vi "Send Control Drag Starting.vi"(0 "Message Enqueuer in":refnum<class "Message Enqueuer.lvclass">, 1 "Drag Mode":enum32{"copy or move", "copy only", "move only"}(ring), 3 "EventFilter Reference":T3, 5 "CtlRef":refnum<vi>, 7 "Time":u32, 9 "Coords":T2, 11 "Button":u16, 12 "Mods":cluster{"Double Click":bool, "Menu Key":bool}, 13 "PlatMods":T4, 14 "Data":T1(array[cluster])) -> (4 "Filtered EventDataMessage":refnum<class "ControlDragStartingMsg.lvclass">, 15 "error out":errorcluster)   [LabVIEW 2020, in "MVA Framework.lvlib" / "ActorEvents.lvlib" / "ControlDragStartingMsg.lvclass"]
doc: "<License>\nCopyright © 2017 Composed Systems, LLC | All rights reserved\nwww.composed.io\n\nAuthor: Ethan Stern <ethan.stern@composed.io>\n\nThis software is provided \"AS IS\" WITHOUT WARRANTIES, either express or implied, AND IS FOR EDUCATIONAL PURPOSES ONLY.\n</License>"
uses:
  ControlDragStartingMsg.lvclass
  <vilib>/ActorFramework/Message Enqueuer/Message Enqueuer.lvclass
  IEventFilter/EventFilter Reference.ctl
  IEventFilter/IEventFilter.lvclass
  <vilib>/Utility/miscctls.llb/LVPoint32TypeDef.ctl
  ControlDragStartingMsg.lvclass/ControlDragStartingMsg.ctl
  EventDataMessage/EventDataMessage.lvclass/EventDataMessage.ctl
  <vilib>/ActorFramework/Message Enqueuer/Message Enqueuer.lvclass/Message Enqueuer.ctl
  <vilib>/ActorFramework/Message Enqueuer/Enqueue.vi
  <vilib>/Utility/error.llb/Clear Errors.vi
  EventDataMessage/EventDataMessage.lvclass
  C:/Program Files/National Instruments/LabVIEW 2020/vi.lib/ActorFramework/Message/Message.lvclass
  <vilib>/ActorFramework/Message Priority Queue/Priority Enqueue.vi
panel:
  in  "error in (no error)":errorcluster
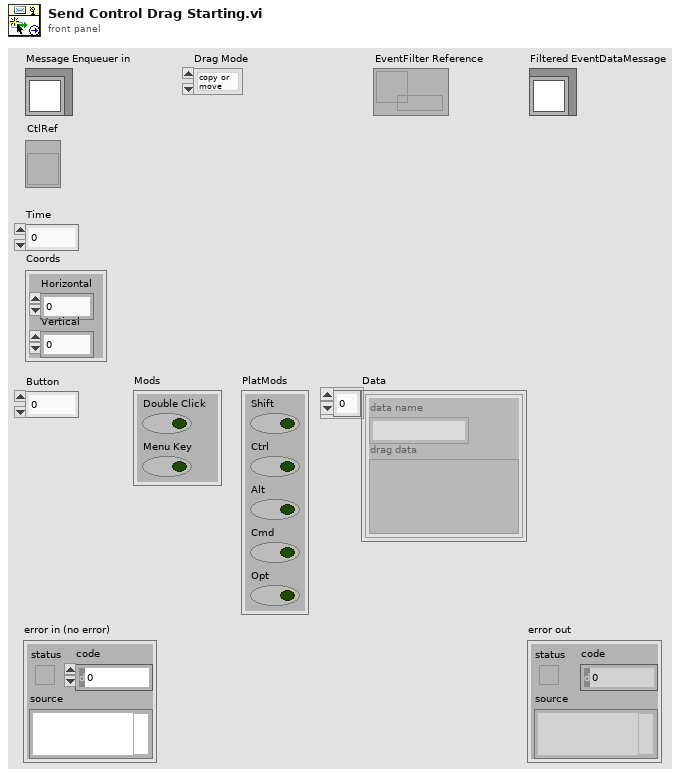
[diagram p1: front panel]
types:
  T1 = cluster{"data name":string, "drag data":variant}[]
  T2 = typedef "LVPoint32TypeDef.ctl" = cluster{"Horizontal":i32, "Vertical":i32}
  T3 = typedef "MVA Framework.lvlib/ActorEvents.lvlib/IEventFilter.lvclass/EventFilter Reference.ctl" = refnum<data-value>
  T4 = cluster{"Shift":bool, "Ctrl":bool, "Alt":bool, "Cmd":bool, "Opt":bool}
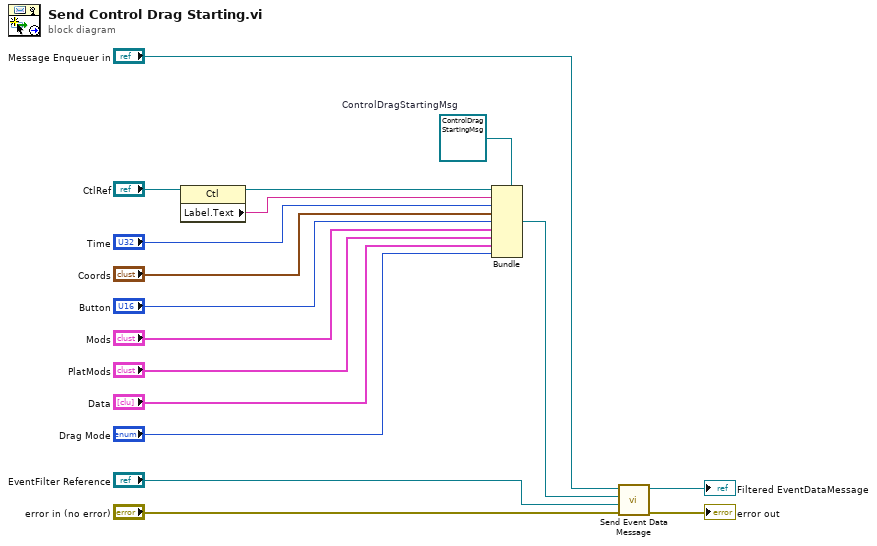
[diagram p0: block diagram]
diagram:
  w17 = refnum<class "ControlDragStartingMsg.lvclass"> refnum  # ControlDragStartingMsg
  n1 = property class="Ctl"(reference="CtlRef") -> (reference out=w11:refnum<vi>, "Label.Text"=w10:string)  [unwired: 1 in, 1 out]
  n2 = Bundle(cluster=w17, w11, w10, "Time", "Coords", "Button", "Mods", "PlatMods", "Data", "Drag Mode") -> (w14:refnum<class "ControlDragStartingMsg.lvclass">)
  n3 = call "Send Event Data Message.vi"("error in (no error)"="error in (no error)", "EventFilter Reference"="EventFilter Reference", "EventDataMessage"=w14, "Message Enqueuer in"="Message Enqueuer in") -> ("error out"=→"error out":errorcluster, "Filtered EventDataMessage"=→"Filtered EventDataMessage":refnum<class "ControlDragStartingMsg.lvclass">)  [unwired: 6 in]
